vi "Service Cycle FG.vi"(8 "Error In":errorcluster, 10 "Cycle Knob":T1(ring), 11 "Action":T2=enum."Get") -> (0 "Error Out":errorcluster, 3 "Cycle Knob Out":T1(ring))   [LabVIEW 2016]
uses:
  type defs/Service Mode Pointer.ctl
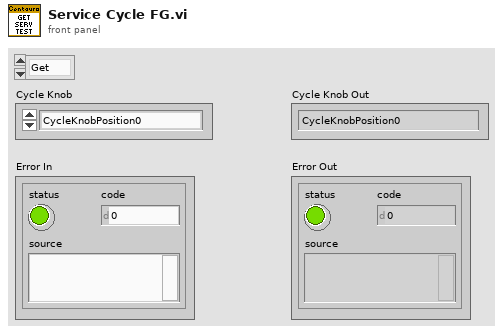
[diagram p1: front panel]
types:
  T1 = enum16{"CycleKnobPosition0", "CycleKnobPosition1", "CycleKnobPosition2", "CycleKnobPosition3", "CycleKnobPosition4", "CycleKnobPosition5", "CycleKnobPosition6", "CycleKnobPosition7", "CycleKnobPosition8", "CycleKnobPosition9", "CycleKnobPosition10", "CycleKnobPosition11"}
  T2 = typedef "Service Mode Pointer.ctl" = enum16{"Set ", "Get"}
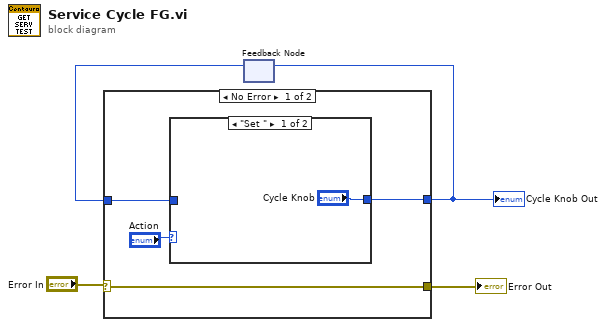
[diagram p0: block diagram]
diagram:
  n1 = feedback #1() -> (w2:T1)  [unwired: 1 in]
  n2 = case shown="No Error" "Error In" {
    selector: "Error In" -> [w7 w12]
    tunnel: [w7 w12] -> w3
    tunnel: [w6 w11] -> w1
    tunnel: w2 -> [w5 w11]
    frame No Error {
      n3 = case shown="\"Set \"" "Action" {
        tunnel: ["Cycle Knob" w10] -> w6
        tunnel: w5 -> [_ w10]
        frame "Set " {
        }
        frame "Get", Default {
        }
      }
    }
    frame Error {
    }
  }
  "Error Out" <- w3
  "Cycle Knob Out" <- w1
  n4 = feedback-in #1(w1) -> ()
